vi "Example-DigitalINSimple.vi"() -> ()   [LabVIEW 2018]
panel:
  out "backsize out":i32
  in  "Fall":u32=255 format="%.0x"
  in  "Rais":u32=255 format="%.0x"
  in  "Channel":u32=255 format="%.0x"
  out "Frequency(Hz)":i32=40000000
  out "Scope Graph":cluster{dbl[], i32[]}(graph) caption="XY图"
  in  "trigcond":enum16{"Raising", "Falling", "Either"}(ring)
  in  "trigsrc":T1(ring)
  in  "trigtype":enum16{"edge", "pulse", "trasition"}(ring)
  in  "timeout":i32
  in  "buffersize":i32=2048
  out "returns":i32[](array[numeric])
  in  "Div":i32=1
  out "error out":errorcluster caption="错误输出"
  in  "error in (no error)":errorcluster caption="错误输入（无错误）"
  out "ftHandle out":u64=363562184
  in  "设备索引":i32
  # "0x0FFF"
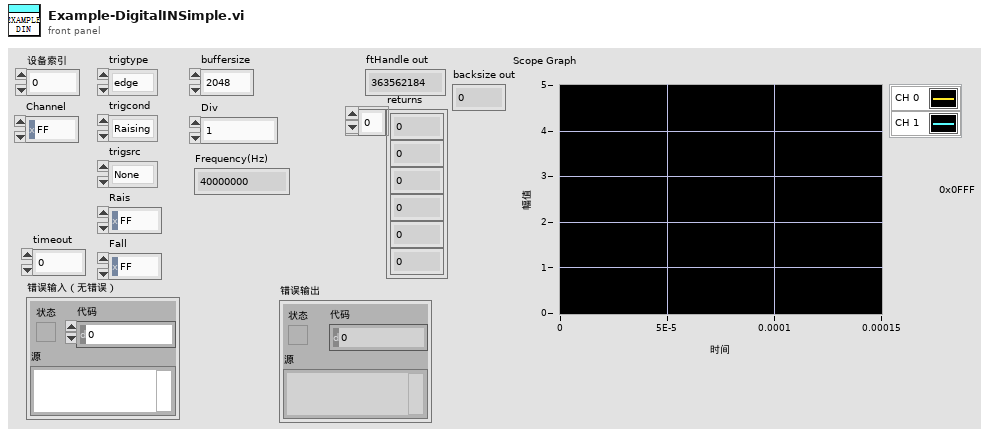
[diagram p1: front panel]
types:
  T1 = enum16{"None", "DetectorAnalogInCH1", "DetectorAnalogInCH2", "AnalogOut1", "AnalogOut2", "DetectorDigitalIn", "DigitalOut", "Manule", "External 1", "External 2", "DigitalIn"}
  T2 = enum16{"CLIFFStateReady", "CLIFFStateArmed", "CLIFFStateDone", "CLIFFStateRunning", "CLIFFStateConfig", "CLIFFStatePrefill", "CLIFFStateTriggered", "CLIFFStateWait"}
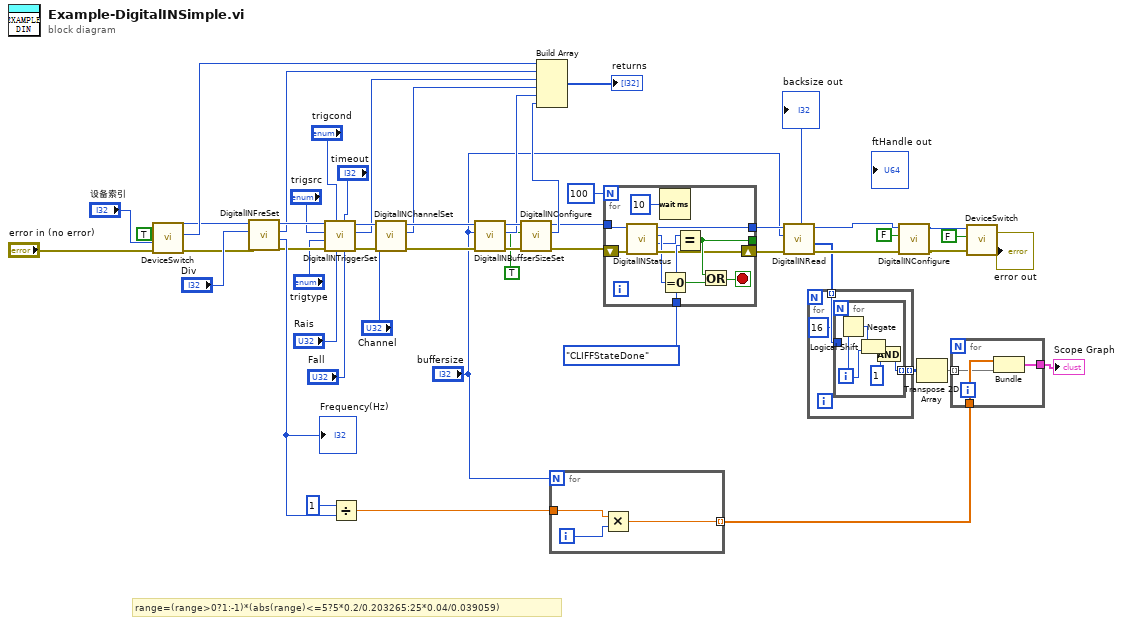
[diagram p0: block diagram]
diagram:
  # "range=(range>0?1:-1)*(abs(range)<=5?5*0.2/0.203265:25*0.04/0.039059)"
  n1 = call "DeviceSwitch.vi"("error in (no error)"="error in (no error)", "Device Index"="设备索引", "Open"=TRUE) -> ("error out"=w30:errorcluster, "function return"=w44:i32, "handle out"=w39:u64)  [unwired: 4 in, 2 out]
  n2 = call "DigitalINFreSet.vi"("error in (no error)"=w30, "div"="Div", "handle"=w39) -> ("error out"=w31:errorcluster, "Frequency(Hz)"=w41:i32, "function return"=w29:i32, "handle out"=w38:u64)  [unwired: 5 in]
  "Frequency(Hz)" <- w41
  n3 = call "DigitalINTriggerSet.vi"("Fall"="Fall", "timeout"="timeout", "Rais"="Rais", "trigcond"="trigcond", "error in (no error)"=w31, "trigtype"="trigtype", "trigsrc"="trigsrc", "handle"=w38) -> ("error out"=w32:errorcluster, "function return"=w28:i32, "handle out"=w37:u64)  [unwired: 1 in]
  n4 = Divide(x=1, y=w41) -> (x/y=w48:dbl)
  n5 = call "DigitalINChannelSet.vi"("error in (no error)"=w32, "Channel"="Channel", "handle"=w37) -> ("error out"=w33:errorcluster, "function return"=w27:i32, "handle out"=w36:u64)  [unwired: 6 in]
  n6 = call "DigitalINBuffserSizeSet.vi"("error in (no error)"=w33, "BufferSize"="buffersize", "handle"=w36) -> ("error out"=w34:errorcluster, "function return"=w26:i32, "handle out"=w35:u64)  [unwired: 6 in]
  n7 = call "DigitalINConfigure.vi"("error in (no error)"=w34, "enable"=TRUE, "handle"=w35) -> ("error out"=w24:errorcluster, "function return"=w25:i32, "handle out"=w23:u64)  [unwired: 6 in]
  n8 = Build Array(w44, w29, w28, w27, w26, w25) -> (→"returns":i32[])
  n9 = for {
    N: "buffersize" -> [_]
    tunnel: w48 -> [w54]
    tunnel: [w53] -> w4 mode=indexing
    i -> [w55]
    n10 = Multiply(x=w54, y=w55) -> (x*y=w53:dbl)
  }
  n11 = for {
    N: 100 -> [_]
    shift-right: [w58] -> w10
    shift-left: w24 -> [w61]
    tunnel: T2."CLIFFStateDone" ("ANIStatus") -> [w66]
    tunnel: [w59] -> w11
    tunnel: [w65] -> _
    tunnel: w23 -> [w60]
    stop <- w63 stop-if-true
    n12 = call "DigitalINStatus.vi"("error in (no error)"=w61, "handle"=w60) -> ("error out"=w58:errorcluster, "status"=w56:i32, "function return"=w57:i32, "handle out"=w59:u64)  [unwired: 6 in]
    n13 = Wait (ms)(milliseconds to wait=u32 10 ("等待时间（毫秒）")) -> ()  [unwired: 1 out]
    n14 = Equal To 0?(x=w57) -> (x = 0?=w62:bool)
    n15 = Equal?(x=w56, y=w66) -> (x = y?=w65:bool)
    n16 = Or(x=w65, y=w62) -> (x .or. y?=w63:bool)
  }
  n17 = call "DigitalINRead.vi"("error in (no error)"=w10, "size"="buffersize", "handle"=w11) -> ("error out"=w9:errorcluster, "RxBuffer out"=w5:u16[], "handle out"=w6:u64, "backsize out"=→"backsize out":i32)  [unwired: 4 in, 1 out]
  n18 = for {
    tunnel: w5 -> [w69] mode=indexing
    tunnel: [w68] -> w2 mode=indexing
    n19 = for {
      N: 16 -> [_]
      tunnel: w69 -> [_]
      tunnel: [w73] -> w68 mode=indexing
      i -> [w71]
      n20 = Negate(x=w71) -> (-x=w70:i32)
      n21 = Logical Shift(y=w70, x=w71) -> (x << y=w74:i32)
      n22 = And(x=w74, y=1) -> (x .and. y?=w73:i32)
    }
  }
  n23 = call "DigitalINConfigure.vi"("error in (no error)"=w9, "enable"=FALSE ("Run"), "handle"=w6) -> ("error out"=w14:errorcluster, "handle out"=w13:u64)  [unwired: 6 in, 1 out]
  n24 = Transpose 2D Array(2D array=w2) -> (transposed array=w1:i32[][])
  n25 = for {
    tunnel: [w77] -> w3
    tunnel: w4 -> [w76]
    tunnel: w1 -> [w75] mode=indexing
    n26 = Bundle(w76, w75) -> (w77:cluster{dbl[], i32[]})  [unwired: 1 in]
  }
  "Scope Graph" <- w3
  n27 = call "DeviceSwitch.vi"("error in (no error)"=w14, "Open"=FALSE, "handle"=w13) -> ("error out"=→"error out":errorcluster)  [unwired: 4 in, 4 out]
